vi "DMM-Read-Voltage-rev1.vi"() -> ()   [LabVIEW 2020]
doc: "This example shows how to select a function, use a trigger delay, and read multiple measurements. It also shows how to calculate the timeout for multiple measurements based on the trigger delay and the number of points."
uses:
  <instrlib>/ke2000/KE2000/ke2000 Configure Measurement.vi
panel:
  out "progress bar":u8(slide) scale=0.0..100.0
  in  "Test Duration":T1(ring)
  out "error out":errorcluster
  out "Voltage/Time (Discharge chart)":dbl[](graph)
  in  "error in":errorcluster
  in  "Function (0: DC Volts)":u16(ring) items=["DC Volts", "AC Volts", "DC Current", "AC Current", "2-Wire Resistance", "4-Wire Resistance"]
  in  "VISA resource name":refnum<visa-resource-name>="DMM1"
  out "Units":string[](array[string])
  out "Data":dbl[](array[numeric])
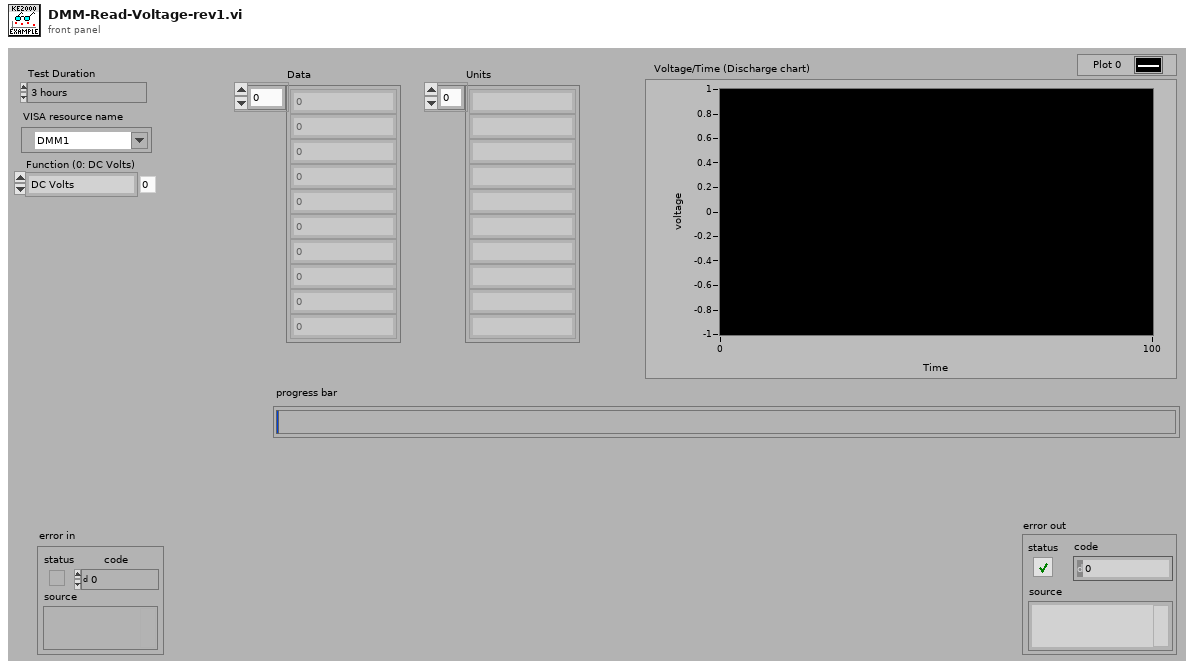
[diagram p1: front panel]
types:
  T1 = enum16{"3 hours", "6 hours", "12 hours", "24 hours", "2 days", "3 days", "4 days", "5 days", "6 days", "7 days"}
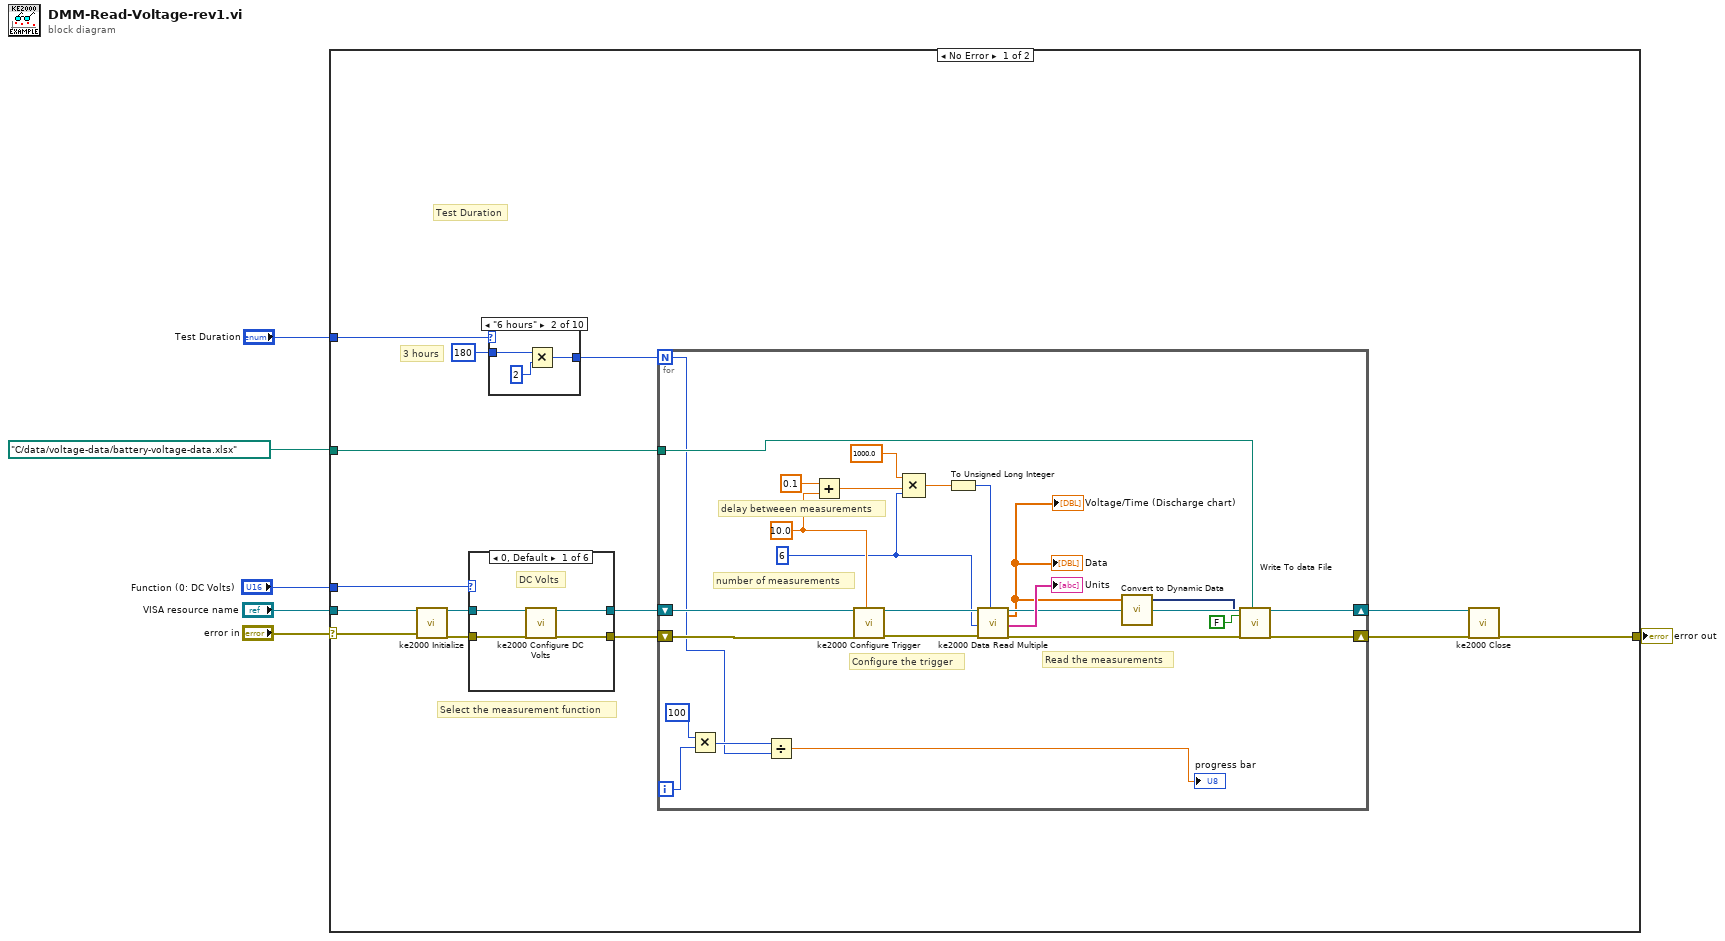
[diagram p0: block diagram]
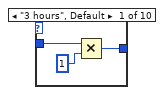
[diagram p2: hidden frame]
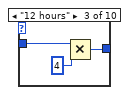
[diagram p3: hidden frame]
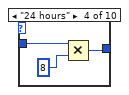
[diagram p4: hidden frame]
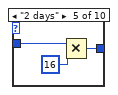
[diagram p5: hidden frame]
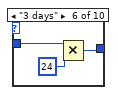
[diagram p6: hidden frame]
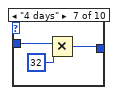
[diagram p7: hidden frame]
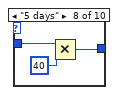
[diagram p8: hidden frame]
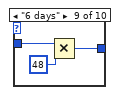
[diagram p9: hidden frame]
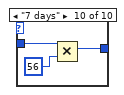
[diagram p10: hidden frame]
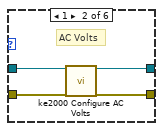
[diagram p11: hidden frame]
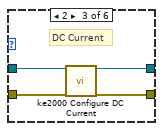
[diagram p12: hidden frame]
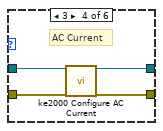
[diagram p13: hidden frame]
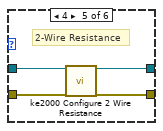
[diagram p14: hidden frame]
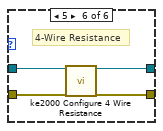
[diagram p15: hidden frame]
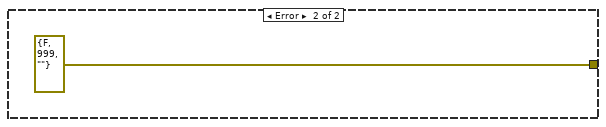
[diagram p16: hidden frame]
diagram:
  n1 = case shown="No Error" "error in" {
    selector: "error in" -> [w13 _]
    tunnel: "VISA resource name" -> [w19 _]
    tunnel: "Function (0: DC Volts)" -> [w18 _]
    tunnel: [w12 errorcluster {"status"=FALSE, "code"=999, "source"=""} ("error out")] -> w3
    tunnel: path "C:/data/voltage-data/battery-voltage-data.xlsx" ("Filename") -> [w11 _]
    tunnel: "Test Duration" -> [w9 _]
    frame No Error {
      # "3 hours"
      # "Test Duration"
      # "Select the measurement function"
      n2 = call <instrlib>:"ke2000 Initialize.vi"("VISA resource name"=w19, "error in (no error)"=w13) -> ("VISA resource name out"=w14:refnum<visa-resource-name>, "error out"=w15:errorcluster)  [unwired: 16 in]
      n3 = case shown="0, Default" w18 {
        tunnel: w15 -> [w78 w82 w86 w90 w94 w98]
        tunnel: w14 -> [w77 w81 w85 w89 w93 w97]
        tunnel: [w76 w80 w84 w88 w92 w96] -> w16
        tunnel: [w75 w79 w83 w87 w91 w95] -> w17
        frame 0, Default {
          # "DC Volts"
          n4 = call-poly <instrlib>:"ke2000 Configure DC Volts.vi"("VISA resource name"=w77, "error in (no error)"=w78) -> ("VISA resource name out"=w75:refnum<visa-resource-name>, "error out"=w76:errorcluster)  [unwired: 16 in]
        }
        frame 1 {
          # "AC Volts"
          n5 = call-poly <instrlib>:"ke2000 Configure AC Volts.vi"("VISA resource name"=w81, "error in (no error)"=w82) -> ("VISA resource name out"=w79:refnum<visa-resource-name>, "error out"=w80:errorcluster)  [unwired: 16 in]
        }
        frame 2 {
          # "DC Current"
          n6 = call-poly <instrlib>:"ke2000 Configure DC Current.vi"("VISA resource name"=w85, "error in (no error)"=w86) -> ("VISA resource name out"=w83:refnum<visa-resource-name>, "error out"=w84:errorcluster)  [unwired: 16 in]
        }
        frame 3 {
          # "AC Current"
          n7 = call-poly <instrlib>:"ke2000 Configure AC Current.vi"("VISA resource name"=w89, "error in (no error)"=w90) -> ("VISA resource name out"=w87:refnum<visa-resource-name>, "error out"=w88:errorcluster)  [unwired: 16 in]
        }
        frame 4 {
          # "2-Wire Resistance"
          n8 = call-poly <instrlib>:"ke2000 Configure 2 Wire Resistance.vi"("VISA resource name"=w93, "error in (no error)"=w94) -> ("VISA resource name out"=w91:refnum<visa-resource-name>, "error out"=w92:errorcluster)  [unwired: 16 in]
        }
        frame 5 {
          # "4-Wire Resistance"
          n9 = call-poly <instrlib>:"ke2000 Configure 4 Wire Resistance.vi"("VISA resource name"=w97, "error in (no error)"=w98) -> ("VISA resource name out"=w95:refnum<visa-resource-name>, "error out"=w96:errorcluster)  [unwired: 16 in]
        }
      }
      n10 = case shown="\"6 hours\"" w9 {
        tunnel: 180 -> [w23 w25 w28 w31 w34 w37 w40 w42 w46 w49]
        tunnel: [w21 w24 w27 w30 w33 w36 w39 w43 w45 w48] -> w7
        frame "3 hours", Default {
          n11 = Multiply(x=w23, y=1) -> (x*y=w21:i32)
        }
        frame "6 hours" {
          n12 = Multiply(x=w25, y=2) -> (x*y=w24:i32)
        }
        frame "12 hours" {
          n13 = Multiply(x=w28, y=4) -> (x*y=w27:i32)
        }
        frame "24 hours" {
          n14 = Multiply(x=w31, y=8) -> (x*y=w30:i32)
        }
        frame "2 days" {
          n15 = Multiply(x=w34, y=16) -> (x*y=w33:i32)
        }
        frame "3 days" {
          n16 = Multiply(x=w37, y=24) -> (x*y=w36:i32)
        }
        frame "4 days" {
          n17 = Multiply(x=w40, y=32) -> (x*y=w39:i32)
        }
        frame "5 days" {
          n18 = Multiply(x=w42, y=40) -> (x*y=w43:i32)
        }
        frame "6 days" {
          n19 = Multiply(x=w46, y=48) -> (x*y=w45:i32)
        }
        frame "7 days" {
          n20 = Multiply(x=w49, y=56) -> (x*y=w48:i32)
        }
      }
      n21 = for {
        N: w7 -> [w52]
        tunnel: w11 -> [w62]
        shift-right: [w73] -> w20
        shift-left: w17 -> [w65]
        shift-right: [w60] -> w10
        shift-left: w16 -> [w56]
        i -> [w55]
        w57 = 6 ("Number of Readings (10)")
        w58 = 10.0 ("Delay (0 s)")
        # "number of measurements"
        # "delay betweeen measurements"
        # "Read the measurements"
        # "Configure the trigger"
        n22 = Multiply(x=100, y=w55) -> (x*y=w53:i32)
        n23 = Divide(x=w53, y=w52) -> (x/y=→"progress bar":dbl)
        n24 = Add(x=0.1, y=w58) -> (x+y=w67:dbl)
        n25 = call <instrlib>:"ke2000 Configure Trigger.vi"("VISA resource name"=w65, "error in (no error)"=w56, "Delay (0 s)"=w58) -> ("VISA resource name out"=w72:refnum<visa-resource-name>, "error out"=w71:errorcluster)  [unwired: 15 in]
        n26 = Compound Arithmetic op=MULTIPLY(1000.0 ("x"), w67, w57) -> (w66:dbl)
        n27 = To Unsigned Long Integer(number=w66) -> (unsigned 32bit integer=w69:u32)
        n28 = call <instrlib>:"ke2000 Data Read Multiple.vi"("VISA resource name"=w72, "Number of Readings (100)"=w57, "error in (no error)"=w71, "Timeout (25000 ms)"=w69) -> ("VISA resource name out"=w73:refnum<visa-resource-name>, "Data"=w64:dbl[], "Units"=→"Units":string[], "error out"=w61:errorcluster)  [unwired: 11 in, 1 out]
        "Data" <- w64
        "Voltage/Time (Discharge chart)" <- w64
        n29 = call "Convert to Dynamic Data"("Array"=w64) -> ("Dynamic Data Type"=w63:dynamicdata)  [unwired: 3 in]
        n30 = call "Write To data File"("Signals"=w63, "Reset"=FALSE, "error in (no error)"=w61, "Filename"=w62) -> ("error out"=w60:errorcluster)  [unwired: 13 in, 2 out]
      }
      n31 = call <instrlib>:"ke2000 Close.vi"("VISA resource name"=w20, "error in (no error)"=w10) -> ("error out"=w12:errorcluster)  [unwired: 17 in]
    }
    frame Error {
    }
  }
  "error out" <- w3
